vi "Test_output_fixed.vi"() -> ()   [LabVIEW 2013]
uses:
  <vilib>/userdefined/High Color/nirio_resource_hc.ctl
  <vilib>/measure/maspectr.llb/Power Spectrum and PSD Export Mode.ctl
  <vilib>/measure/maspectr.llb/FFT Power Spectrum and PSD for 1 Chan.vi
  <vilib>/FPGAPlugInAG/PXIe-7975R/niLvFpga_Open_PXIe-7975R.vi
  <vilib>/rvi/interface/common/dynamic/niFpgaDynamicAddResources.vi
  <vilib>/FPGAPlugInAG/Dynamic/niLvFpga_Close_Dynamic.vi
  <vilib>/rvi/interface/nirviOpenFPGA/nirviOpenFPGA.xnode
  FPGA Bitfiles/FPGAoutputfixed375_MHz_KcNSHvogqos.lvbitx
  FPGA Bitfiles/FPGAoutputfixed125_MHz_nv4b6Zp6nDA.lvbitx
  <vilib>/rvi/interface/nirviCloseFPGA/nirviCloseFPGA.xnode
  <vilib>/measure/NI_MAPro.lvlib
panel:
  in  "User Data 1":u8=64
  in  "Clock Source":T1(ring)=enum."Internal Clock PLL On (IoModSyncClk)"
  out "power spectrum":cluster{"f0":dbl, "df":dbl, "magnitude":dbl[]}(graph)
  in  "stop":bool
  in  "Ring":u16(ring) items=["125 MHz", "375 MHz"]
  out "Configured?":bool
  out "Clocking Option Configured?":bool
  in  "resource name":T2="RIO0"
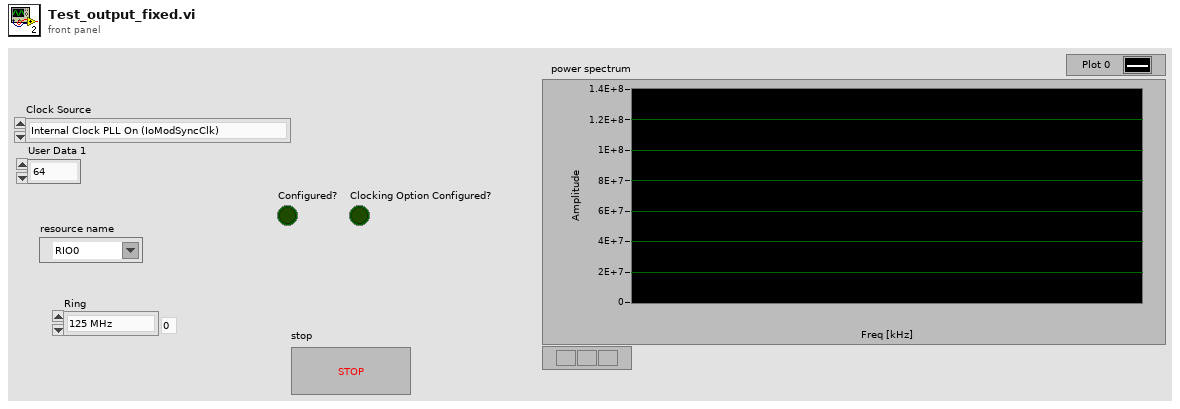
[diagram p1: front panel]
types:
  T1 = enum8{"Internal Clock PLL Off", "Internal Clock PLL On (REF IN)", "External Clock (CLK_IN)", "Internal Clock PLL On (IoModSyncClk)"}
  T2 = typedef "nirio_resource_hc.ctl" = tag
  T3 = typedef "NI_MAPro.lvlib/Power Spectrum and PSD Export Mode.ctl" = u16
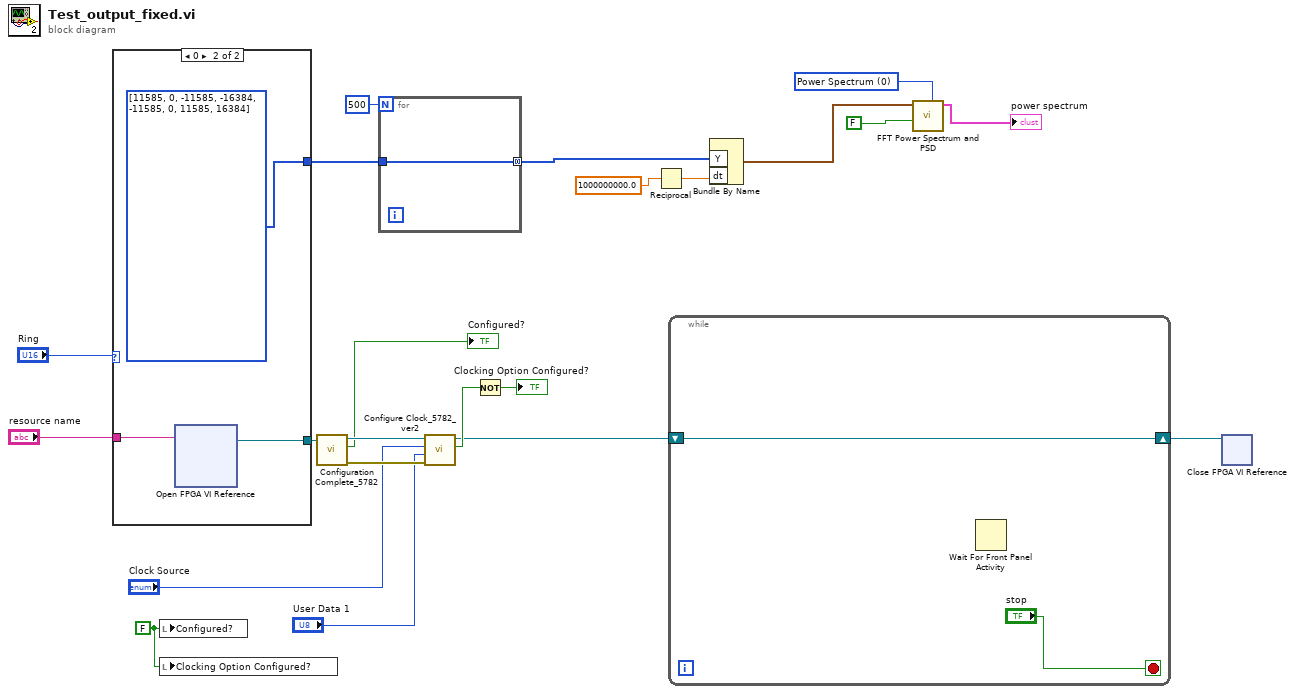
[diagram p0: block diagram]
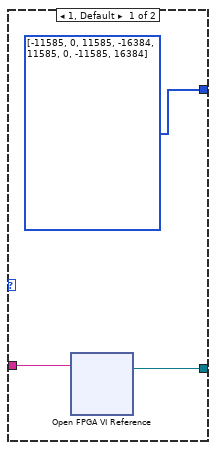
[diagram p2: hidden frame]
diagram:
  w1 = FALSE ("Configured?")
  w8 = T3 0 items=["Power Spectrum", "Power Spectral Density"] ("export mode")
  n1 = case shown="0" "Ring" {
    tunnel: "resource name" -> [w25 w28]
    tunnel: [w24 w27] -> w16
    tunnel: [i16[] [-11585, 0, 11585, -16384, 11585, 0, -11585, 16384] ("output array 2") i16[] [11585, 0, -11585, -16384, -11585, 0, 11585, 16384] ("output array 2")] -> w9
    frame 1, Default {
      n2 = xnode "Open FPGA VI Reference"("resource name"=w25) -> ("FPGA VI Reference Out"=w24:refnum<k20>)  [unwired: 1 in, 1 out]
    }
    frame 0 {
      n3 = xnode "Open FPGA VI Reference"("resource name"=w28) -> ("FPGA VI Reference Out"=w27:refnum<k20>)  [unwired: 1 in, 1 out]
    }
  }
  n4 = local write "Configured?"(w1) -> ()
  n5 = local write "Clocking Option Configured?"(w1) -> ()
  n6 = call "Configuration Complete_5782.vi"("FPGA VI Reference in"=w16) -> ("error out"=w21:errorcluster, "Configured?"=→"Configured?":bool, "FPGA VI Reference out"=w20:refnum<k20>)  [unwired: 8 in]
  n7 = for {
    N: 500 -> [_]
    tunnel: [w29] -> w2 mode=concatenating
    tunnel: w9 -> [w29]
  }
  n8 = call "Configure Clock_5782_ver2.vi"("error in"=w21, "User Data 1"="User Data 1", "Clock Source"="Clock Source", "FPGA VI Reference"=w20) -> ("Configuration Error"=w14:bool, "FPGA VI Reference out"=w12:refnum<k20>)  [unwired: 5 in, 1 out]
  n9 = Not(x=w14) -> (.not. x?=→"Clocking Option Configured?":bool)
  n10 = Reciprocal(x=1000000000.0 ("dt")) -> (1/x=w4:dbl)
  n11 = while {
    shift-right: [w31] -> w11
    shift-left: w12 -> [w31]
    stop <- "stop" stop-if-true
    n12 = Wait For Front Panel Activity() -> ()  [unwired: 3 in, 1 out]
  }
  n13 = Bundle By Name("Y"=w2, "dt"=w4) -> (w7:waveform(i16))  [unwired: 1 in]
  n14 = call-poly <vilib>:"FFT Power Spectrum and PSD.vi"("export mode"=w8, "dB On (F)"=FALSE, "time signal"=w7) -> ("Power Spectrum / PSD"=→"power spectrum":cluster{"f0":dbl, "df":dbl, "magnitude":dbl[]})  [unwired: 5 in, 3 out]
  n15 = xnode "Close FPGA VI Reference"("FPGA VI Reference In"=w11) -> ()  [unwired: 1 in, 1 out]
